vi "Graphics-Set Plot Colors.vi"(0 "XY Graph":refnum<vi>, 7 "Color Box":u32(colorbox), 11 "error in (no error)":errorcluster) -> (15 "error out":errorcluster)   [LabVIEW 2020]
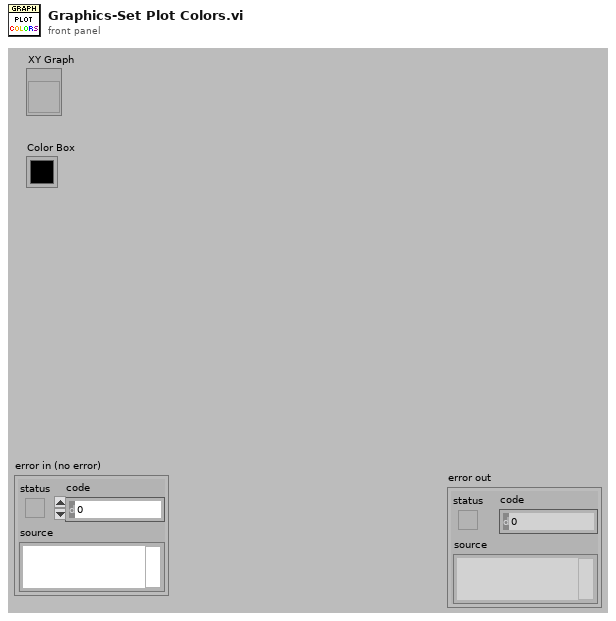
[diagram p1: front panel]
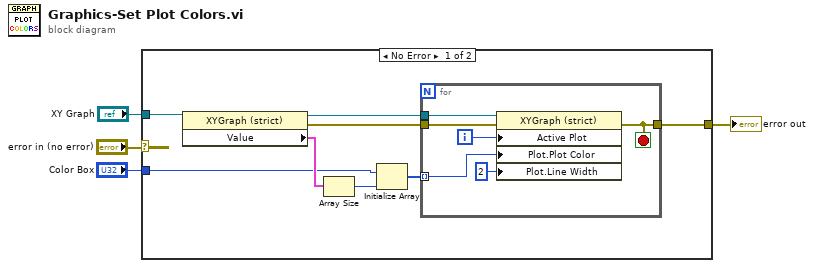
[diagram p0: block diagram]
diagram:
  n1 = case shown="No Error" "error in (no error)" {
    selector: "error in (no error)" -> [_ w19]
    tunnel: "XY Graph" -> [w12 _]
    tunnel: "Color Box" -> [w7 _]
    tunnel: [w5 w19] -> w1
    frame No Error {
      n2 = property class="XYGraph (strict)"(reference=w12) -> (reference out=w11:refnum<vi>, error out=w10:errorcluster, "Value"=w9:cluster{"Frequency":dbl[], "Frequency":dbl[]}[])  [unwired: 1 in]
      n3 = Array Size(array=w9) -> (size(s)=w8:i32)
      n4 = Initialize Array(w7, w8) -> (w6:u32[])
      n5 = for {
        tunnel: w11 -> [w18]
        tunnel: w10 -> [w17]
        tunnel: w6 -> [w15] mode=indexing
        tunnel: [w14] -> w5
        i -> [w16]
        stop <- w14 stop-if-true
        n6 = property class="XYGraph (strict)"(reference=w18, error in=w17, "Active Plot"=w16, "Plot.Plot Color"=w15, "Plot.Line Width"=u8 2) -> (error out=w14:errorcluster)  [unwired: 1 out]
      }
    }
    frame Error {
    }
  }
  "error out" <- w1
